vi "get wavefront in array form.vi"(8 "error in (no error)":errorcluster, 11 "HasoSlopes in":refnum<class "HasoSlopes.lvclass">) -> (0 "error out":errorcluster, 1 "Phase out":refnum<class "Phase.lvclass">, 2 "data":sgl[][](array[numeric]), 3 "Pupil out":refnum<class "Pupil.lvclass">, 4 "StatisticsData":T1, 5 "HasoData out":refnum<class "HasoData.lvclass">, 7 "ComputePhaseSet.lvclass 2":refnum<class "ComputePhaseSet.lvclass">)   [LabVIEW 2020, in "HASO4_3.lvclass"]
uses:
  HASO4_3.lvclass
  WaveKit/Classes/HasoSlopes/HasoSlopes.lvclass
  WaveKit/Classes/ComputePhaseSet/ComputePhaseSet.lvclass
  WaveKit/Classes/HasoData/HasoData.lvclass
  WaveKit/Classes/Pupil/Pupil.lvclass
  WaveKit/Classes/Phase/Phase.lvclass
  WaveKit/Controls/StatisticsData.ctl
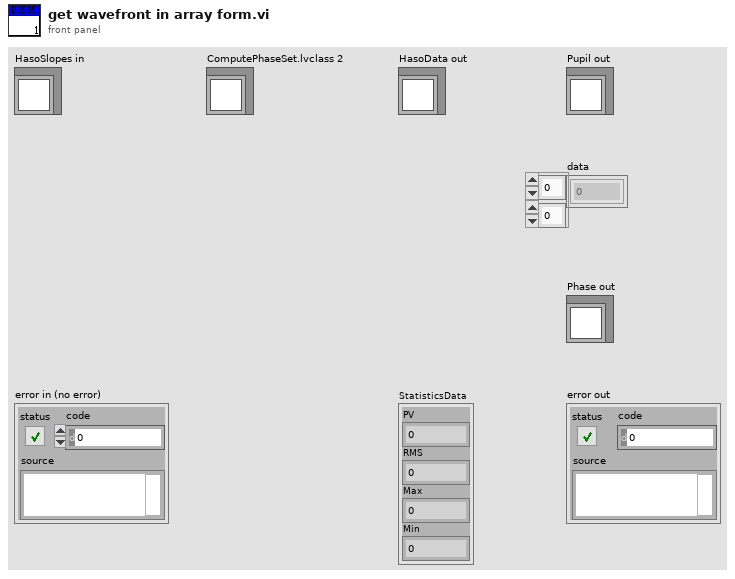
[diagram p1: front panel]
types:
  T1 = typedef "StatisticsData.ctl" = cluster{"PV":sgl, "RMS":dbl, "Max":sgl, "Min":sgl}
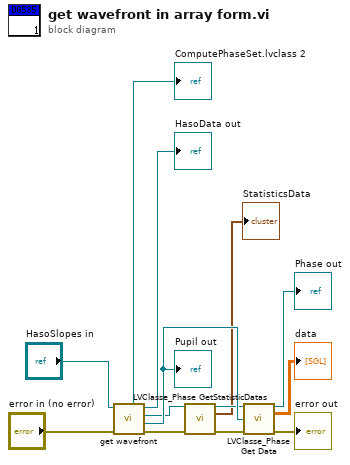
[diagram p0: block diagram]
diagram:
  n1 = call "get wavefront.vi"("error in"="error in (no error)", "HasoSlopes in"="HasoSlopes in") -> ("error out"=w5:errorcluster, "Pupil (new)"=w8:refnum<class "Pupil.lvclass">, "Phase"=w4:refnum<class "Phase.lvclass">, "HasoData out"=→"HasoData out":refnum<class "HasoData.lvclass">, "ComputePhaseSet.lvclass 2"=→"ComputePhaseSet.lvclass 2":refnum<class "ComputePhaseSet.lvclass">)  [unwired: 5 in]
  "Pupil out" <- w8
  n2 = call "LVClasse_Phase GetStatisticDatas.vi"("Phase in"=w4, "error in (no error)"=w5) -> ("Phase out"=w3:refnum<class "Phase.lvclass">, "StatisticsData"=→"StatisticsData":T1, "error out"=w2:errorcluster)  [unwired: 11 in]
  n3 = call "LVClasse_Phase Get Data.vi"("Phase in"=w3, "Pupil"=w8, "error in (no error)"=w2) -> ("Phase out"=→"Phase out":refnum<class "Phase.lvclass">, "data"=→"data":sgl[][], "error out"=→"error out":errorcluster)  [unwired: 9 in, 1 out]
